vi "ModelProcess.vi"(8 "error in (no error)":errorcluster, 11 "Data In":T1) -> (0 "error out":errorcluster, 3 "Data Out":T1)   [LabVIEW 2013]
uses:
  controls/Data.ctl
panel:
  # "日期"
  # "機種名稱"
  # "機種代號"
  # "商品條碼"
  # "OK"
  # "台"
  # "NG"
  # "總計"
  # "台"
  # "日期"
  # "機種名稱"
  # "機種代號"
  # "商品條碼"
  # "OK"
  # "台"
  # "NG"
  # "總計"
  # "台"
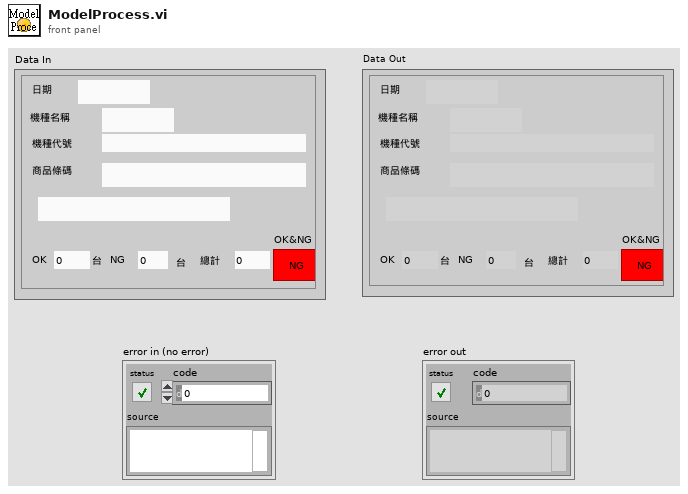
[diagram p1: front panel]
types:
  T1 = typedef "Data.ctl" = cluster{"Date":string, "BarCode1":string, "BarCode2":string, "BarCode3":string, "Message":string, "OK Count":u16, "NG Count":u16, "Total Count":u16, "ModelData":string[][], "OK&NG":bool, "COM1":refnum<visa-resource-name>, "COM2":refnum<visa-resource-name>, "IO":i32}
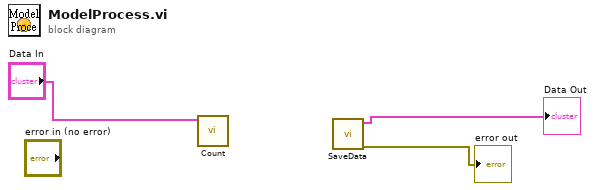
[diagram p0: block diagram]
diagram:
  n1 = call "Count.vi"("Data In"="Data In") -> ()  [unwired: 10 in, 1 out]
  n2 = call "SaveData.vi"() -> ("error out"=→"error out":errorcluster, "Data Out"=→"Data Out":T1)  [unwired: 10 in]
